vi "SPI_Example_Port Code_kyles.vi"(10 "Port":u8, 11 "FPGA IO":T1={"SCLK"="DIO18", "CS_1"="DIO16", "MOSI"="DIO26", "MISO"="DIO25"}) -> ()   [LabVIEW 2012]
uses:
  Code/FPGA SPI_Globals.vi
  <vilib>/rvi/LocalResourceManager/LocalResourceManager.xnode
  Controls/FPGA SPI_Port Loop State.ctl
  <vilib>/Platform/TimedLoop/XDataNode/wakeup.ctl
  <vilib>/Platform/TimedLoop/XDataNode/XDNodeRunTimeDep.lvlib
  <vilib>/Platform/TimedLoop/XDataNode/nitl_modes.ctl
  <vilib>/Platform/TimedLoop/XDataNode/timing_clust.ctl
  <vilib>/Platform/TimedLoop/XDataNode/XDataNode.xnode
  Controls/FPGA SPI_SPI Loop State.ctl
  <vilib>/eio/EIONode/EIONode.xnode
  <vilib>/rvi/DataTransferAndStorage/Container/XNode/niFpgaContainer.xnode
  <vilib>/rvi/DataTransferAndStorage/Container/Common/niFpgaContainerMetaDataKey.ctl
  <vilib>/rvi/DataTransferAndStorage/Container/Common/niFpgaContainerInitializationParameters.ctl
  <vilib>/rvi/DataTransferAndStorage/Container/Common/niFpgaTransferTypeControl.ctl
  <vilib>/rvi/DataTransferAndStorage/Container/Common/niFpgaContainerArbitrationOptionsControl.ctl
  <vilib>/rvi/DataTransferAndStorage/Container/Common/niFpgaContainerImplementationControl.ctl
  <vilib>/rvi/DataTransferAndStorage/Container/Common/niFpgaDataTypeControl.ctl
  <vilib>/rvi/DataTransferAndStorage/Container/Common/niFpgaContainerState.ctl
  <vilib>/rvi/DataTransferAndStorage/Container/Common/niFpgaContainerSetEmuInfo.vi
  <vilib>/rvi/eio/common/nirviEmuReportErrorAndStop.vi
  <vilib>/rvi/DataTransferAndStorage/Container/Common/niFpgaContainerGetUniqueNameForEmu.vi
  <vilib>/rvi/FIFO/Fifo_Types/niFpgaFifoControlLogicControl.ctl
  <vilib>/rvi/Memory/Memory_Types/niFpgaMemoryInterfaceConfiguration.ctl
  <vilib>/rvi/FIFO/Fifo_Resource/nirvififoEmulationRead.vi
  <vilib>/rvi/FIFO/Fifo_Resource/nirvififoEmulationWrite.vi
  <vilib>/rvi/eio/common/nirviEmuTemplateMethod_errors.vi
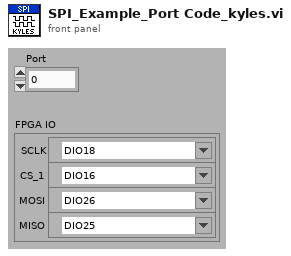
[diagram p1: front panel]
types:
  T1 = cluster{"SCLK":refnum<k21>, "CS_1":refnum<k21>, "MOSI":refnum<k21>, "MISO":refnum<k21>}
  T2 = cluster{"CS":u8, "CS Active State":bool, "CPOL":bool, "CPHA":bool, "Wait Ticks":u32, "Read?":bool}
  T3 = typedef "FPGA SPI_Port Loop State.ctl" = enum8{"Idle", "Start", "Configure Hardware", "Start Hardware", "Set Done", "Wait Until Done", "Restart Port"}
  T4 = typedef "FPGA SPI_SPI Loop State.ctl" = enum8{"Initialize", "Set CS", "Read From FIFO", "Send Byte", "Write to FIFO", "Reset CS", "Read Delay"}
  T5 = typedef "XDNodeRunTimeDep.lvlib/timing_clust.ctl" = cluster{"Expected End [f-1]":u64, "Actual End [f-1]":u64, "Finished Late? [f-1]":bool, "Expected End [i-1]":u64, "Actual End [i-1]":u64, "Finished Late? [i-1]":bool, "Expected Start [i]":u64, "Actual Start [i]":u64, "Expected Start [f]":u64, "Actual Start [f]":u64, "Source Name":string, "Structure Name":string, "Period":i64, "Deadline":i64, "Offset":i64, "Start":i64, "Priority":i32, "Timeout":i32, "Mode":T6, "Wakeup Reason":T7, "Error":errorcluster, "Source Type":string, "Secondary Source Type":string, "Global End Time":u64, "Global Start Time":u64, "Frame Duration":u64, "Iteration Duration":u64, "Assigned CPU":i32, "I/O Scan Engine Mode":u32}
  T6 = typedef "XDNodeRunTimeDep.lvlib/nitl_modes.ctl" = enum32{"No Change", "Process missed periods, maintain original phase", "Discard missed periods, maintain original phase", "Process missed periods, ignore original phase", "Discard missed periods, ignore original phase"}
  T7 = typedef "XDNodeRunTimeDep.lvlib/wakeup.ctl" = enum32{"Normal", "Aborted", "Asynchronous wakeup", "Timing source error", "Timed loop error", "Timeout"}
  T8 = typedef "FPGA SPI_Cmd.ctl" = enum8{"Idle", "Write/Read SPI", "Configure", "Restart"}
  T9 = cluster{"MOSI":bool[], "MISO":bool[], "MOSI Byte Index":i8, "MISO Byte Index":i8}
  T10 = cluster{"Next State":T4, "Wait Count":u32, "Total Bits":u16, "Current Bit":u16, "Total Bytes":u16, "Scots Sate":T4, "Scotts Wait":u32, "CS Reset Wait":u32}
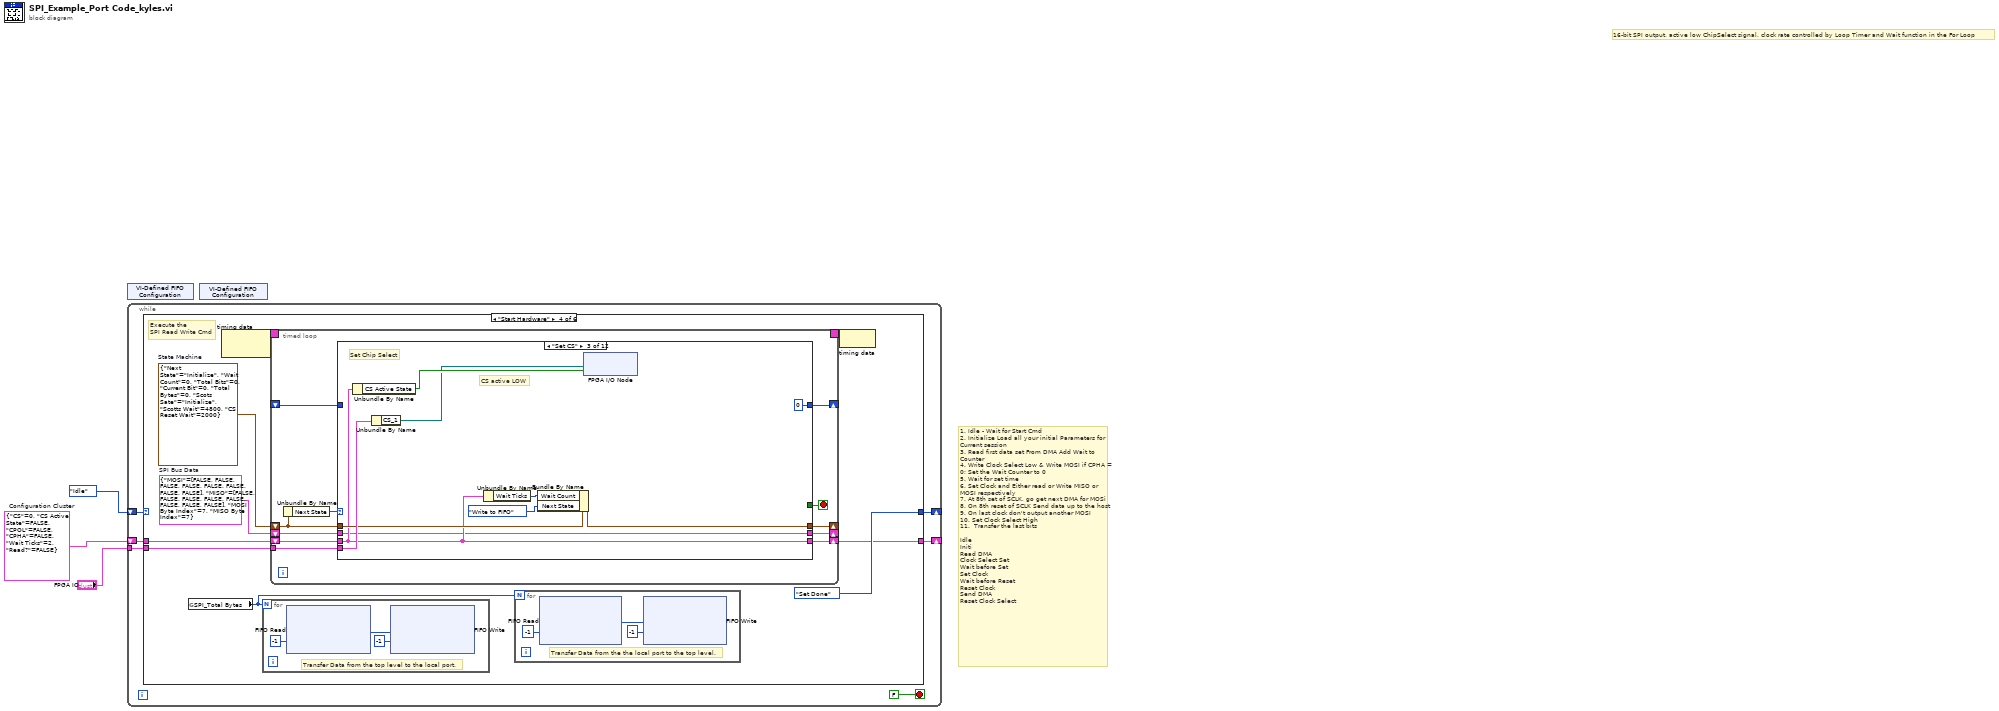
[diagram p0: block diagram]
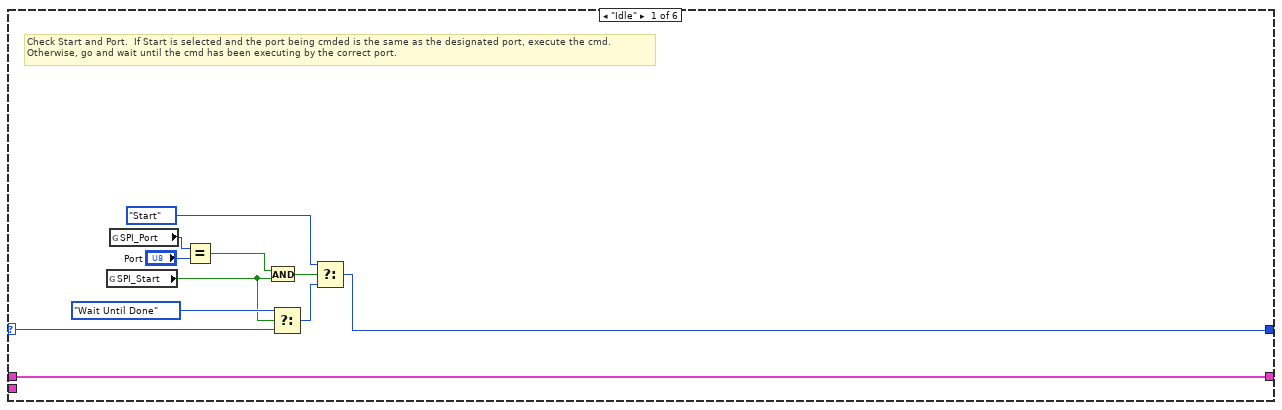
[diagram p2: hidden frame]
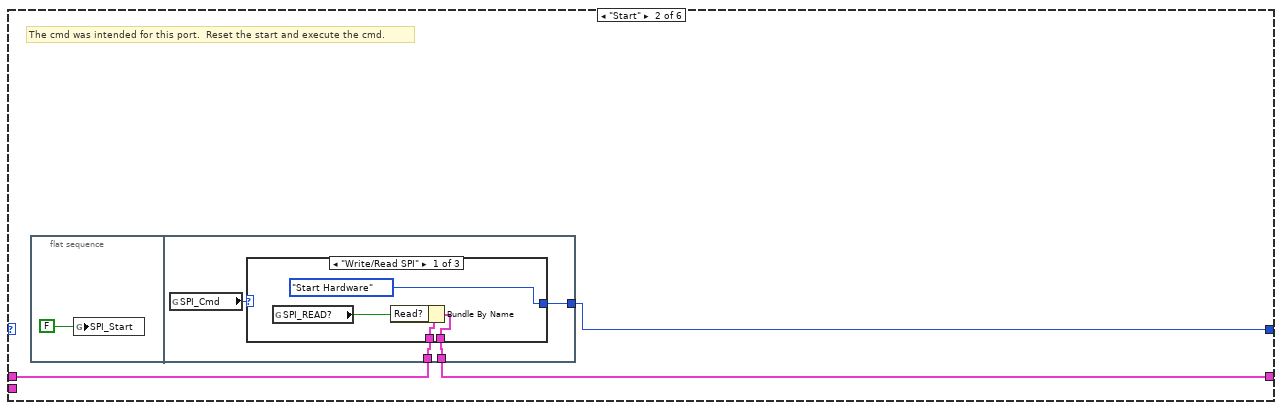
[diagram p3: hidden frame]
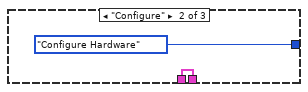
[diagram p4: hidden frame]
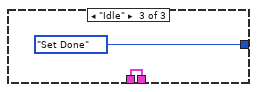
[diagram p5: hidden frame]
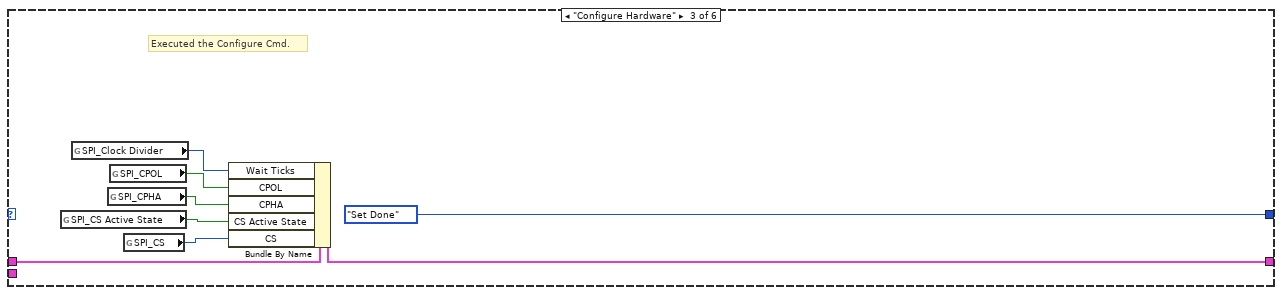
[diagram p6: hidden frame]
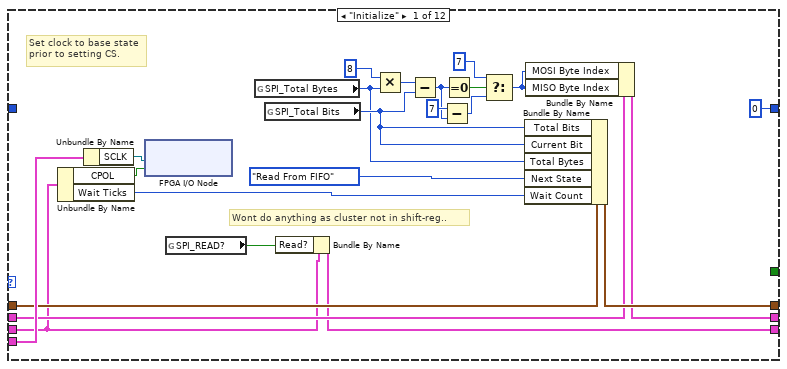
[diagram p7: hidden frame]
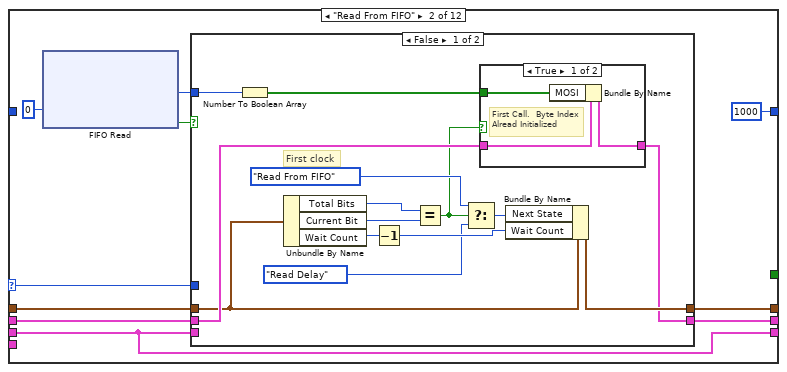
[diagram p8: hidden frame]
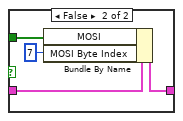
[diagram p9: hidden frame]
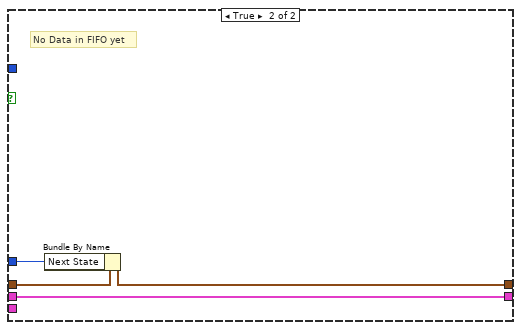
[diagram p10: hidden frame]
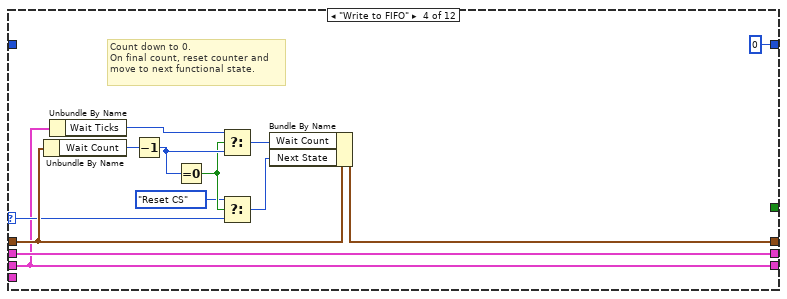
[diagram p11: hidden frame]
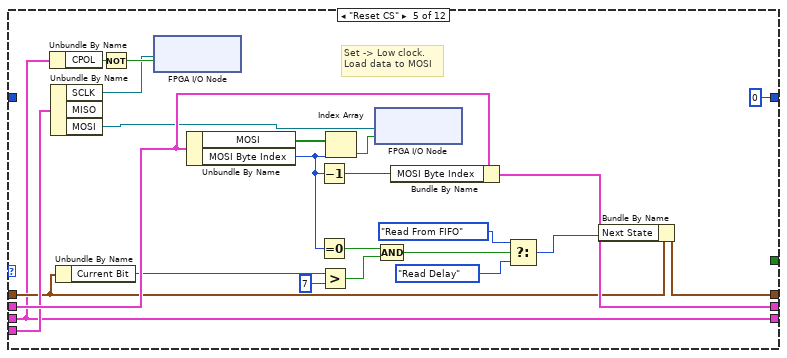
[diagram p12: hidden frame]
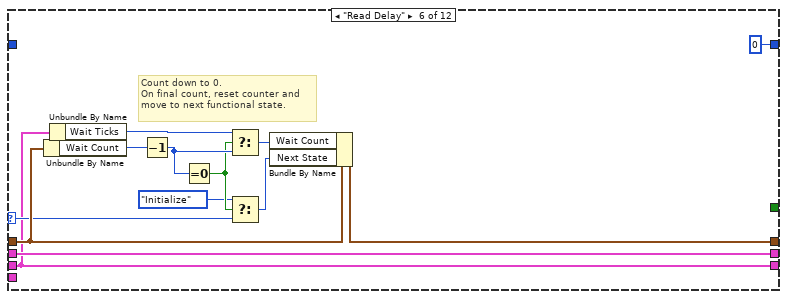
[diagram p13: hidden frame]
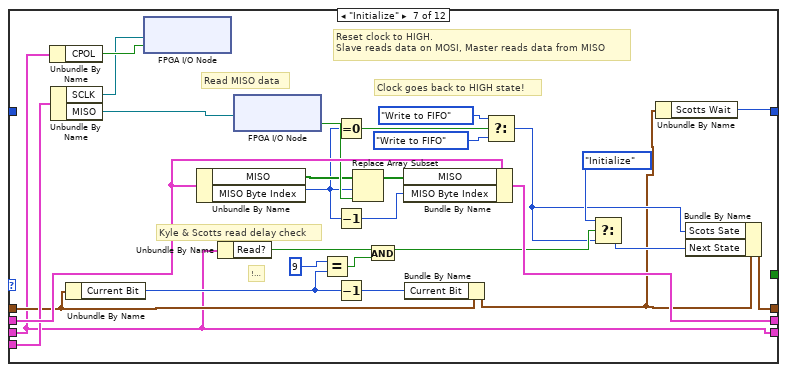
[diagram p14: hidden frame]
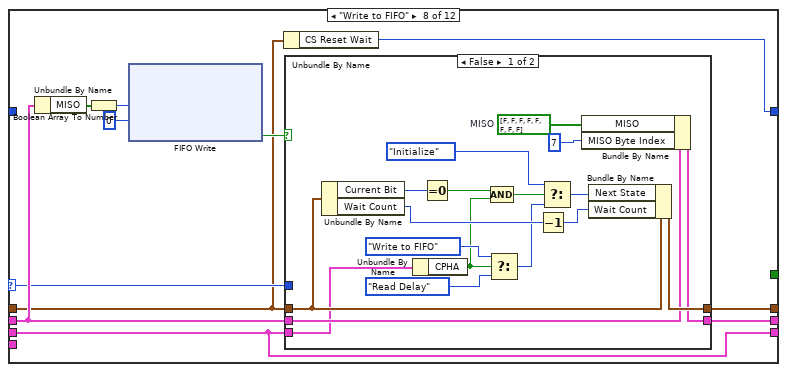
[diagram p15: hidden frame]
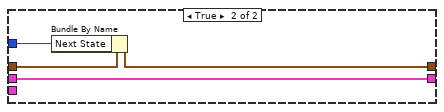
[diagram p16: hidden frame]
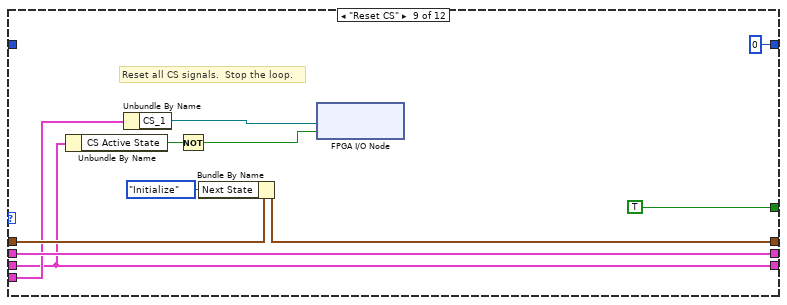
[diagram p17: hidden frame]
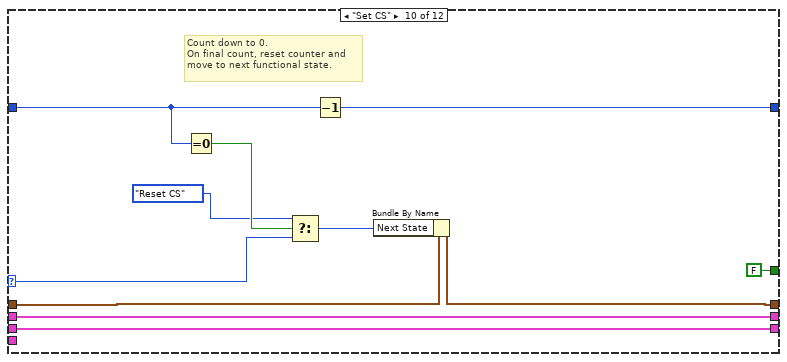
[diagram p18: hidden frame]
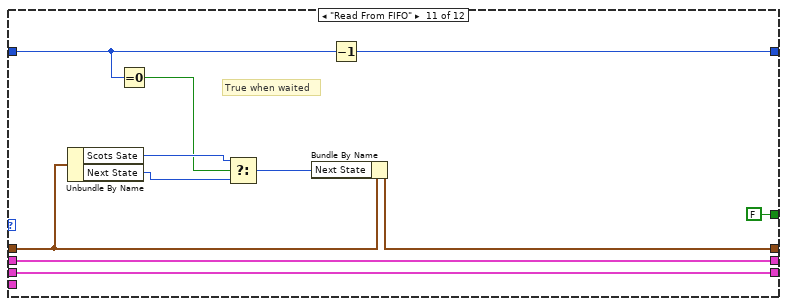
[diagram p19: hidden frame]
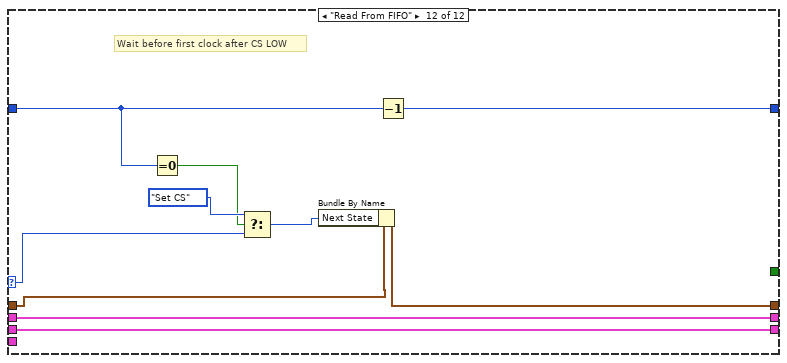
[diagram p20: hidden frame]
diagram:
  w2 = T2 {"CS"=0, "CS Active State"=FALSE, "CPOL"=FALSE, "CPHA"=FALSE, "Wait Ticks"=2, "Read?"=FALSE}  # Configuration Cluster
  # "16-bit SPI output, active low ChipSelect signal, clock rate controlled by Loop Timer and Wait function in the For Loop"
  # "1. Idle - Wait for Start Cmd\n2. Initialize Load all your initial Parameters for Current session\n3. Read first data set From DMA Add Wait to Counter\n4. Write Clock Select Low & Write MOSI if CPHA = 0; Set the Wait Counter to 0\n5. Wait for set time\n6. Set Clock and Either read or Write MISO or MOSI respectively\n7. At 8th set of SCLK, go get next DMA for MOSi\n8. On 8th reset of SCLK Send data up to the host\n9. On last clock don't output another MOSI\n10. Set Clock Select High \n11.  Transfer the last bits\n\nIdle\nIniti\nRead DMA\nClock Select Set\nWait before Set\nSet Clock\nWait before Reset\nReset Clock\nSend DMA\nReset Clock Select"
  n1 = xnode "VI-Defined FIFO Configuration"() -> ()  [unwired: 1 out]
  n2 = while {
    shift-right: [w8] -> _
    shift-left: FPGA_SPI_Port_Loop_State."Idle" ("Action") -> [w7]
    shift-right: [w4] -> _
    shift-left: w2 -> [w6]
    tunnel: "FPGA IO" -> [w5]
    stop <- FALSE stop-if-true
    n3 = case shown="\"Start Hardware\"" w7 {
      selector: w7 -> [w10 _ _ _ _ w301]
      tunnel: [w19 w23 FPGA_SPI_Port_Loop_State."Set Done" ("Action") FPGA_SPI_Port_Loop_State."Set Done" ("Action") FPGA_SPI_Port_Loop_State."Idle" ("Action") w300] -> w8
      tunnel: w6 -> [w14 w22 w40 w45 w296 w299]
      tunnel: w5 -> [_ _ _ w50 _ _]
      tunnel: [w14 w21 w39 w46 w296 w299] -> w4
      frame "Idle" {
        # "Check Start and Port.  If Start is selected and the port being cmded is the same as the designated port, execute the cmd.\nOtherwise, go and wait until the cmd has been executing by the correct port."
        n4 = global read "FPGA SPI_Globals.vi" "SPI_Start"() -> (w11:bool)
        n5 = global read "FPGA SPI_Globals.vi" "SPI_Port"() -> (w18:u8)
        n6 = Equal?(x=w18, y="Port") -> (x = y?=w12:bool)
        n7 = And(x=w12, y=w11) -> (x .and. y?=w16:bool)
        n8 = Select(t=FPGA_SPI_Port_Loop_State."Wait Until Done" ("Action"), s=w11, f=w10) -> (s? t:f=w15:T3)
        n9 = Select(t=FPGA_SPI_Port_Loop_State."Start" ("Action"), s=w16, f=w15) -> (s? t:f=w19:T3)
      }
      frame "Start" {
        # "The cmd was intended for this port.  Reset the start and execute the cmd."
        n10 = flat-sequence {
          tunnel: [w27] -> w23
          tunnel: [w26] -> w21
          tunnel: w22 -> [w25]
          frame #0 {
            n11 = global write "FPGA SPI_Globals.vi" "SPI_Start"(FALSE ("Write Flag")) -> ()
          }
          frame #1 {
            n12 = global read "FPGA SPI_Globals.vi" "SPI_Cmd"() -> (w28:T8)
            n13 = case shown="\"Write/Read SPI\"" w28 {
              tunnel: [FPGA_SPI_Port_Loop_State."Start Hardware" ("Action") FPGA_SPI_Port_Loop_State."Configure Hardware" ("Action") FPGA_SPI_Port_Loop_State."Set Done" ("Action")] -> w27
              tunnel: [w30 w33 w35] -> w26
              tunnel: w25 -> [w29 w33 w35]
              frame "Write/Read SPI" {
                n14 = global read "FPGA SPI_Globals.vi" "SPI_READ?"() -> (w31:bool)
                n15 = Bundle By Name(cluster=w29, "Read?"=w31) -> (w30:T2)
              }
              frame "Configure" {
              }
              frame "Idle" {
              }
            }
          }
        }
      }
      frame "Configure Hardware" {
        # "Executed the Configure Cmd."
        n16 = global read "FPGA SPI_Globals.vi" "SPI_CS Active State"() -> (w42:bool)
        n17 = global read "FPGA SPI_Globals.vi" "SPI_Clock Divider"() -> (w37:u32)
        n18 = global read "FPGA SPI_Globals.vi" "SPI_CPHA"() -> (w41:bool)
        n19 = global read "FPGA SPI_Globals.vi" "SPI_CPOL"() -> (w44:bool)
        n20 = global read "FPGA SPI_Globals.vi" "SPI_CS"() -> (w43:u8)
        n21 = Bundle By Name(cluster=w40, "Wait Ticks"=w37, "CPOL"=w44, "CPHA"=w41, "CS Active State"=w42, "CS"=w43) -> (w39:T2)
      }
      frame "Start Hardware" {
        w48 = T9 {"MOSI"=[FALSE, FALSE, FALSE, FALSE, FALSE, FALSE, FALSE, FALSE], "MISO"=[FALSE, FALSE, FALSE, FALSE, FALSE, FALSE, FALSE, FALSE], "MOSI Byte Index"=7, "MISO Byte Index"=7}  # SPI Bus Data
        w49 = T10 {"Next State"=enum."Initialize", "Wait Count"=0, "Total Bits"=0, "Current Bit"=0, "Total Bytes"=0, "Scots Sate"=enum."Initialize", "Scotts Wait"=4800, "CS Reset Wait"=2000}  # State Machine
        # "Execute the \nSPI Read Write Cmd"
        n22 = global read "FPGA SPI_Globals.vi" "SPI_Total Bytes"() -> (w47:u16)
        n23 = node-c288() -> (w52:T5)  [unwired: 1 out]
        n24 = for {
          N: w47 -> [_]
          # "Transfer Data from the top level to the local port."
          n25 = xnode ("FIFO Read")("Timeout"=-1) -> ("Element"=w58:u8)  [unwired: 1 in, 2 out]
          n26 = xnode ("FIFO Write")("Element"=w58, "Timeout"=-1) -> ()  [unwired: 1 in, 2 out]
        }
        n27 = timed-loop {
          timing-out: [_] -> w51
          timing: w52 -> [_]
          shift-right: [w70] -> _
          shift-left: w49 -> [w69]
          shift-right: [w66] -> _
          shift-left: w48 -> [w67]
          tunnel: w50 -> [w64]
          shift-right: [w61] -> _
          shift-left: _ -> [w62]
          shift-right: [w60] -> w46
          shift-left: w45 -> [w63]
          stop <- w65 stop-if-true
          n28 = Unbundle By Name(w69) -> ("Next State"=w68:T4)
          n29 = case shown="\"Set CS\"" w68 {
            selector: w68 -> [_ w96 _ w144 _ w179 _ w219 _ w260 _ w288]
            tunnel: w69 -> [w90 w98 w136 w150 w166 w186 w208 w218 w258 w268 w279 w285]
            tunnel: [w89 w101 w138 w151 w174 w187 w215 w224 w259 w267 w280 w287] -> w70
            tunnel: w63 -> [w73 w94 w130 w139 w152 w175 w188 w216 w249 w262 w271 w284]
            tunnel: w67 -> [w76 w99 w129 w142 w170 w184 w213 w222 w256 w270 w281 w286]
            tunnel: [w79 w100 w129 w142 w171 w184 w212 w221 w256 w270 w281 w286] -> w66
            tunnel: w64 -> [w93 _ w137 _ w169 _ w211 _ w254 _ _ _]
            tunnel: [_ _ _ _ _ _ _ _ TRUE ("Start Hardware") FALSE ("Start Hardware") FALSE ("Start Hardware") _] -> w65
            tunnel: w62 -> [_ _ _ _ _ _ _ _ _ w265 w274 w283]
            tunnel: [u32 0 ("Scotts Wait") u32 1000 ("Scotts Wait") u32 0 ("Scotts Wait") u32 0 ("Scotts Wait") u32 0 ("Scotts Wait") u32 0 ("Scotts Wait") w190 w217 u32 0 ("Scotts Wait") w266 w275 w282] -> w61
            tunnel: [w72 w94 w130 w139 w152 w175 w188 w216 w249 w262 w271 w284] -> w60
            frame "Initialize" {
              # "Wont do anything as cluster not in shift-reg.."
              # "Set clock to base state\nprior to setting CS."
              n30 = Unbundle By Name(w73) -> ("CPOL"=w91:bool, "Wait Ticks"=w75:u32)
              n31 = Unbundle By Name(w93) -> ("SCLK"=w92:refnum<k21>)
              n32 = xnode "FPGA I/O Node"("I/O Item"=w91, "FPGA I/O In"=w92) -> ()  [unwired: 1 out]
              n33 = global read "FPGA SPI_Globals.vi" "SPI_READ?"() -> (w71:bool)
              n34 = global read "FPGA SPI_Globals.vi" "SPI_Total Bytes"() -> (w77:u16)
              n35 = global read "FPGA SPI_Globals.vi" "SPI_Total Bits"() -> (w78:u16)
              n36 = Bundle By Name(cluster=w73, "Read?"=w71) -> (w72:T2)
              n37 = Multiply(x=u16 8 ("y"), y=w77) -> (x*y=w86:u16)
              n38 = Subtract(x=w86, y=w78) -> (x-y=w83:i8)
              n39 = Subtract(x=i8 7, y=w83) -> (x-y=w81:i8)
              n40 = Equal To 0?(x=w83) -> (x = 0?=w82:bool)
              n41 = Select(t=i8 7 ("y"), s=w82, f=w81) -> (s? t:f=w80:i8)
              n42 = Bundle By Name(cluster=w90, "Total Bits"=w78, "Current Bit"=w78, "Total Bytes"=w77, "Next State"=FPGA_SPI_SPI_Loop_State."Read From FIFO", "Wait Count"=w75) -> (w89:T10)
              n43 = Bundle By Name(cluster=w76, "MOSI Byte Index"=w80, "MISO Byte Index"=w80) -> (w79:T9)
            }
            frame "Read From FIFO" {
              n44 = xnode ("FIFO Read")("Timeout"=0) -> ("Element"=w102:u8, "Timed Out?"=w97:bool)  [unwired: 1 in, 1 out]
              n45 = case shown="False" w97 {
                tunnel: w102 -> [w117 _]
                tunnel: [w116 w125] -> w101
                tunnel: [w111 w128] -> w100
                tunnel: w99 -> [w110 w128]
                tunnel: w98 -> [w108 w126]
                tunnel: w94 -> [_ _]
                tunnel: w96 -> [_ w127]
                frame False {
                  # "First clock"
                  n46 = Number To Boolean Array(number=w117) -> (Boolean array=w109:bool[])
                  n47 = Unbundle By Name(w108) -> ("Total Bits"=w113:u16, "Current Bit"=w115:u16, "Wait Count"=w107:u32)
                  n48 = Decrement(x=w107) -> (x-1=w106:u32)
                  n49 = Equal?(x=w113, y=w115) -> (x = y?=w105:bool)
                  n50 = Select(t=FPGA_SPI_SPI_Loop_State."Read From FIFO" ("Next State"), s=w105, f=FPGA_SPI_SPI_Loop_State."Read Delay" ("Next State")) -> (s? t:f=w112:T4)
                  n51 = case shown="True" w105 {
                    tunnel: [w120 w124] -> w111
                    tunnel: w110 -> [w119 w123]
                    tunnel: w109 -> [w118 w122]
                    frame True {
                      # "First Call.  Byte Index Alread Initialized"
                      n52 = Bundle By Name(cluster=w119, "MOSI"=w118) -> (w120:T9)
                    }
                    frame False {
                      n53 = Bundle By Name(cluster=w123, "MOSI"=w122, "MOSI Byte Index"=i8 7) -> (w124:T9)
                    }
                  }
                  n54 = Bundle By Name(cluster=w108, "Next State"=w112, "Wait Count"=w106) -> (w116:T10)
                }
                frame True {
                  # "No Data in FIFO yet"
                  n55 = Bundle By Name(cluster=w126, "Next State"=w127) -> (w125:T10)
                }
              }
            }
            frame "Set CS" {
              # "CS active LOW"
              # "Set Chip Select"
              n56 = Unbundle By Name(w130) -> ("CS Active State"=w133:bool)
              n57 = Unbundle By Name(w137) -> ("CS_1"=w132:refnum<k21>)
              n58 = Unbundle By Name(w130) -> ("Wait Ticks"=w135:u32)
              n59 = Bundle By Name(cluster=w136, "Wait Count"=w135, "Next State"=FPGA_SPI_SPI_Loop_State."Write to FIFO" ("Enum")) -> (w138:T10)
              n60 = xnode "FPGA I/O Node"("I/O Item"=w133, "FPGA I/O In"=w132) -> ()  [unwired: 1 out]
            }
            frame "Write to FIFO" {
              # "Count down to 0.\nOn final count, reset counter and\nmove to next functional state."
              n61 = Unbundle By Name(w150) -> ("Wait Count"=w148:u32)
              n62 = Unbundle By Name(w139) -> ("Wait Ticks"=w141:u32)
              n63 = Decrement(x=w148) -> (x-1=w149:u32)
              n64 = Equal To 0?(x=w149) -> (x = 0?=w147:bool)
              n65 = Select(t=w141, s=w147, f=w149) -> (s? t:f=w146:u32)
              n66 = Select(t=FPGA_SPI_SPI_Loop_State."Reset CS", s=w147, f=w144) -> (s? t:f=w145:T4)
              n67 = Bundle By Name(cluster=w150, "Wait Count"=w146, "Next State"=w145) -> (w151:T10)
            }
            frame "Reset CS" {
              # "Set -> Low clock.\nLoad data to MOSI"
              n68 = Unbundle By Name(w152) -> ("CPOL"=w172:bool)
              n69 = Unbundle By Name(w169) -> ("SCLK"=w167:refnum<k21>, "MOSI"=w168:refnum<k21>)  [unwired: 1 out]
              n70 = Unbundle By Name(w166) -> ("Current Bit"=w165:u16)
              n71 = Not(x=w172) -> (.not. x?=w173:bool)
              n72 = xnode "FPGA I/O Node"("I/O Item"=w173, "FPGA I/O In"=w167) -> ()  [unwired: 1 out]
              n73 = Unbundle By Name(w170) -> ("MOSI"=w163:bool[], "MOSI Byte Index"=w155:i8)
              n74 = Decrement(x=w155) -> (x-1=w154:i8)
              n75 = Equal To 0?(x=w155) -> (x = 0?=w161:bool)
              n76 = Greater?(x=w165, y=u16 7 ("x")) -> (0:w159:bool)
              n77 = Index Array(array=w163, index=w155) -> (element=w162:bool)
              n78 = xnode "FPGA I/O Node"("I/O Item"=w162, "FPGA I/O In"=w168) -> ()  [unwired: 1 out]
              n79 = Compound Arithmetic op=AND(w161, w159) -> (w158:bool)
              n80 = Bundle By Name(cluster=w170, "MOSI Byte Index"=w154) -> (w171:T9)
              n81 = Select(t=FPGA_SPI_SPI_Loop_State."Read From FIFO" ("Enum"), s=w158, f=FPGA_SPI_SPI_Loop_State."Read Delay" ("Enum")) -> (s? t:f=w164:T4)
              n82 = Bundle By Name(cluster=w166, "Next State"=w164) -> (w174:T10)
            }
            frame "Read Delay" {
              # "Count down to 0.\nOn final count, reset counter and\nmove to next functional state."
              n83 = Unbundle By Name(w186) -> ("Wait Count"=w183:u32)
              n84 = Unbundle By Name(w175) -> ("Wait Ticks"=w177:u32)
              n85 = Decrement(x=w183) -> (x-1=w185:u32)
              n86 = Equal To 0?(x=w185) -> (x = 0?=w182:bool)
              n87 = Select(t=w177, s=w182, f=w185) -> (s? t:f=w181:u32)
              n88 = Select(t=FPGA_SPI_SPI_Loop_State."Initialize", s=w182, f=w179) -> (s? t:f=w180:T4)
              n89 = Bundle By Name(cluster=w186, "Wait Count"=w181, "Next State"=w180) -> (w187:T10)
            }
            frame "Initialize" {
              # "Kyle & Scotts read delay check"
              # "!!!!"
              # "Reset clock to HIGH.\nSlave reads data on MOSI, Master reads data from MISO"
              # "Read MISO data"
              # "Clock goes back to HIGH state!"
              n90 = Unbundle By Name(w188) -> ("CPOL"=w214:bool)
              n91 = Unbundle By Name(w211) -> ("SCLK"=w209:refnum<k21>, "MISO"=w210:refnum<k21>)
              n92 = Unbundle By Name(w208) -> ("Current Bit"=w195:u16)
              n93 = xnode "FPGA I/O Node"("I/O Item"=w214, "FPGA I/O In"=w209) -> ()  [unwired: 1 out]
              n94 = Unbundle By Name(w213) -> ("MISO"=w206:bool[], "MISO Byte Index"=w201:i8)
              n95 = Unbundle By Name(w188) -> ("Read?"=w197:bool)
              n96 = xnode "FPGA I/O Node"("FPGA I/O In"=w210) -> ("I/O Item"=w207:bool)  [unwired: 1 out]
              n97 = Equal?(x=u16 9, y=w195) -> (x = y?=w194:bool)
              n98 = Equal To 0?(x=w201) -> (x = 0?=w199:bool)
              n99 = Decrement(x=w201) -> (x-1=w204:i8)
              n100 = Decrement(x=w195) -> (x-1=w200:u16)
              n101 = Replace Array Subset(array=w206, new element=w207, index=w201) -> (w205:bool[])
              n102 = And(x=w197, y=w194) -> (x .and. y?=w196:bool)
              n103 = Bundle By Name(cluster=w213, "MISO"=w205, "MISO Byte Index"=w204) -> (w212:T9)
              n104 = Bundle By Name(cluster=w208, "Current Bit"=w200) -> (w189:T10)
              n105 = Select(t=FPGA_SPI_SPI_Loop_State."Write to FIFO" ("Enum"), s=w199, f=FPGA_SPI_SPI_Loop_State."Write to FIFO" ("Enum")) -> (s? t:f=w191:T4)
              n106 = Select(t=FPGA_SPI_SPI_Loop_State."Initialize" ("Enum"), s=w196, f=w191) -> (s? t:f=w198:T4)
              n107 = Unbundle By Name(w189) -> ("Scotts Wait"=w190:u32)
              n108 = Bundle By Name(cluster=w189, "Scots Sate"=w191, "Next State"=w198) -> (w215:T10)
            }
            frame "Write to FIFO" {
              n109 = Unbundle By Name(w222) -> ("MISO"=w226:bool[])
              n110 = Boolean Array To Number(Boolean array=w226) -> (number=w225:u8)
              n111 = xnode ("FIFO Write")("Element"=w225, "Timeout"=0) -> ("Timed Out?"=w220:bool)  [unwired: 1 in, 1 out]
              n112 = Unbundle By Name(w218) -> ("CS Reset Wait"=w217:u32)
              n113 = case shown="False" w220 {
                tunnel: [w244 w246] -> w224
                tunnel: w218 -> [w243 w247]
                tunnel: w216 -> [w227 _]
                tunnel: w222 -> [w230 w248]
                tunnel: [w228 w248] -> w221
                tunnel: w219 -> [_ w245]
                frame False {
                  w231 = bool[] [FALSE, FALSE, FALSE, FALSE, FALSE, FALSE, FALSE, FALSE]  # MISO
                  n114 = Unbundle By Name(w243) -> ("Current Bit"=w242:u16, "Wait Count"=w239:u32)
                  n115 = Unbundle By Name(w227) -> ("CPHA"=w233:bool)
                  n116 = Equal To 0?(x=w242) -> (x = 0?=w235:bool)
                  n117 = Select(t=FPGA_SPI_SPI_Loop_State."Write to FIFO" ("Next State"), s=w233, f=FPGA_SPI_SPI_Loop_State."Read Delay" ("Next State")) -> (s? t:f=w236:T4)
                  n118 = Compound Arithmetic op=AND(w235, w233) -> (w234:bool)
                  n119 = Decrement(x=w239) -> (x-1=w232:u32)
                  n120 = Select(t=FPGA_SPI_SPI_Loop_State."Initialize" ("Next State"), s=w234, f=w236) -> (s? t:f=w240:T4)
                  n121 = Bundle By Name(cluster=w230, "MISO"=w231, "MISO Byte Index"=i8 7) -> (w228:T9)
                  n122 = Bundle By Name(cluster=w243, "Next State"=w240, "Wait Count"=w232) -> (w244:T10)
                }
                frame True {
                  n123 = Bundle By Name(cluster=w247, "Next State"=w245) -> (w246:T10)
                }
              }
            }
            frame "Reset CS" {
              # "Reset all CS signals.  Stop the loop."
              n124 = Unbundle By Name(w249) -> ("CS Active State"=w255:bool)
              n125 = Unbundle By Name(w254) -> ("CS_1"=w253:refnum<k21>)
              n126 = Not(x=w255) -> (.not. x?=w251:bool)
              n127 = Bundle By Name(cluster=w258, "Next State"=FPGA_SPI_SPI_Loop_State."Initialize" ("Enum")) -> (w259:T10)
              n128 = xnode "FPGA I/O Node"("I/O Item"=w251, "FPGA I/O In"=w253) -> ()  [unwired: 1 out]
            }
            frame "Set CS" {
              # "Count down to 0.\nOn final count, reset counter and\nmove to next functional state."
              n129 = Equal To 0?(x=w265) -> (x = 0?=w264:bool)
              n130 = Select(t=FPGA_SPI_SPI_Loop_State."Reset CS", s=w264, f=w260) -> (s? t:f=w269:T4)
              n131 = Decrement(x=w265) -> (x-1=w266:u32)
              n132 = Bundle By Name(cluster=w268, "Next State"=w269) -> (w267:T10)
            }
            frame "Read From FIFO" {
              # "True when waited"
              n133 = Unbundle By Name(w279) -> ("Scots Sate"=w277:T4, "Next State"=w276:T4)
              n134 = Equal To 0?(x=w274) -> (x = 0?=w273:bool)
              n135 = Select(t=w277, s=w273, f=w276) -> (s? t:f=w278:T4)
              n136 = Bundle By Name(cluster=w279, "Next State"=w278) -> (w280:T10)
              n137 = Decrement(x=w274) -> (x-1=w275:u32)
            }
            frame "Read From FIFO" {
              # "Wait before first clock after CS LOW"
              n138 = Equal To 0?(x=w283) -> (x = 0?=w289:bool)
              n139 = Select(t=FPGA_SPI_SPI_Loop_State."Set CS", s=w289, f=w288) -> (s? t:f=w290:T4)
              n140 = Bundle By Name(cluster=w285, "Next State"=w290) -> (w287:T10)
              n141 = Decrement(x=w283) -> (x-1=w282:u32)
            }
          }
        }
        n142 = for {
          N: w47 -> [_]
          # "Transfer Data from the the local port to the top level."
          n143 = xnode ("FIFO Read")("Timeout"=-1) -> ("Element"=w55:u8)  [unwired: 1 in, 2 out]
          n144 = xnode ("FIFO Write")("Element"=w55, "Timeout"=-1) -> ()  [unwired: 1 in, 2 out]
        }
        n145 = node-c288(w51) -> ()
      }
      frame "Set Done" {
        # "Set the done flag"
        n146 = global write "FPGA SPI_Globals.vi" "SPI_Done"(TRUE ("Done")) -> ()
      }
      frame "Wait Until Done" {
        # "Wait until the executing port finishes."
        n147 = global read "FPGA SPI_Globals.vi" "SPI_Done"() -> (w303:bool)
        n148 = Select(t=FPGA_SPI_Port_Loop_State."Idle" ("Action"), s=w303, f=w301) -> (s? t:f=w300:T3)
      }
    }
  }
  n149 = xnode "VI-Defined FIFO Configuration"() -> ()  [unwired: 1 out]
